vi "CAN Jaguar Config Limits.vi"(6 "Reverse Limit Position":dbl, 8 "error in (no error)":errorcluster, 9 "Forward Limit Position":dbl, 10 "Limit Mode":T1, 11 "CAN Jaguar Ref":T2={"Device Number"=0, "Control Mode"=enum."Percent VBus", "Inverted"=FALSE, "Semaphore"=refnum, "Max Vout"=12.0, "DevStatus"={"status"=FALSE, "code"=0, "source"=""}}) -> (0 "error out":errorcluster, 3 "CAN Jaguar Ref Out":T2={"Device Number"=0, "Control Mode"=enum."Percent VBus", "Inverted"=FALSE, "Semaphore"=refnum, "Max Vout"=12.0, "DevStatus"={"status"=FALSE, "code"=0, "source"=""}})   [LabVIEW 2009, in "CAN.lvlib"]
uses:
  CAN.lvlib
  SubVIs/CAN Motor Message IDs.ctl
  SubVIs/CAN Jaguar Control Mode.ctl
  SubVIs/CAN Jaguar Ref.ctl
  SubVIs/CAN Jaguar Limit Mode.ctl
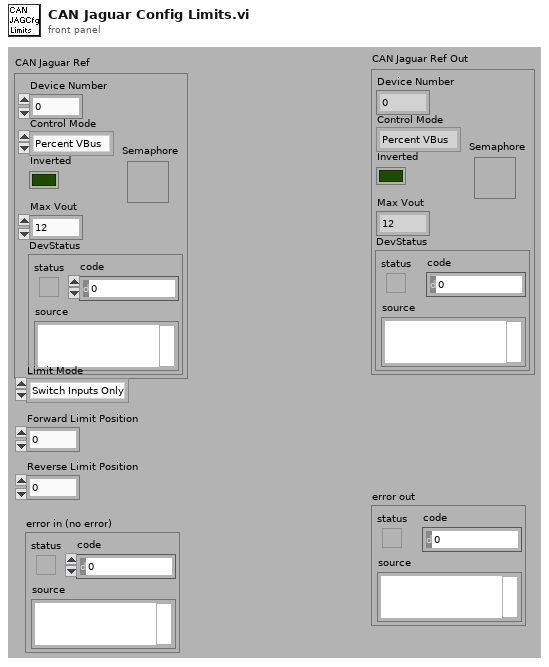
[diagram p1: front panel]
types:
  T1 = typedef "CAN.lvlib/CAN Jaguar Limit Mode.ctl" = enum16{"Switch Inputs Only", "Soft Position Limits"}
  T2 = typedef "CAN.lvlib/CAN Jaguar Ref.ctl" = cluster{"Device Number":u8, "Control Mode":T3, "Inverted":bool, "Semaphore":T4, "Max Vout":dbl, "DevStatus":errorcluster}
  T3 = typedef "CAN.lvlib/CAN Jaguar Control Mode.ctl" = enum16{"Percent VBus", "Speed", "Position", "Current"}
  T4 = typedef "Semaphore RefNum" = refnum<k1>
  T5 = enum16{"big-endian, network order", "native, host order", "little-endian"}
  T6 = typedef "CAN.lvlib/CAN Motor Message IDs.ctl" = u32
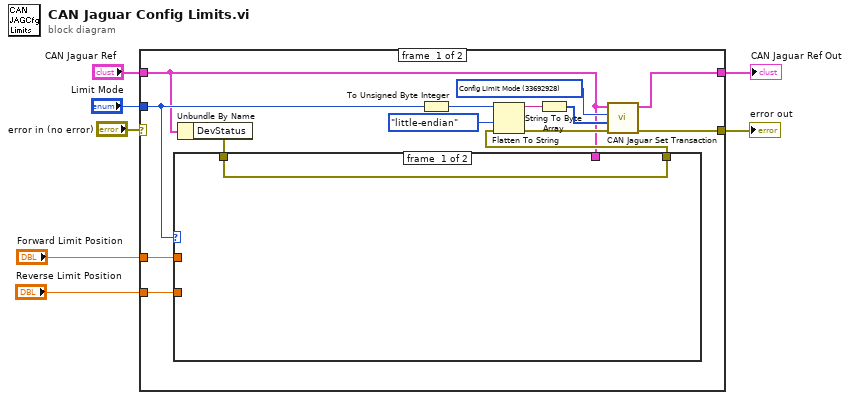
[diagram p0: block diagram]
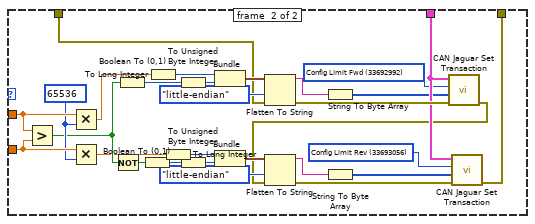
[diagram p2: hidden frame]
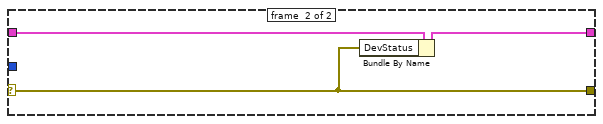
[diagram p3: hidden frame]
diagram:
  n1 = case shown="No Error" "error in (no error)" {
    selector: "error in (no error)" -> [_ w52]
    tunnel: [w11 w52] -> w7
    tunnel: [w12 w53] -> w5
    tunnel: "CAN Jaguar Ref" -> [w8 w54]
    tunnel: "Limit Mode" -> [w18 _]
    tunnel: "Forward Limit Position" -> [w17 _]
    tunnel: "Reverse Limit Position" -> [w16 _]
    frame #0 {
      w9 = T6 33692928 items=["Volt Enable"=33685504, "Volt Disable"=33685568, "Volt Set"=33685632, "Volt Set Ramp"=33685696, "Speed Enable"=33686528, "Speed Disable"=33686592, "Speed Set"=33686656, "Speed P"=33686720, "Speed I"=33686784, "Speed D"=33686848, "Speed Ref"=33686912, "Position Enable"=33688576, "Position Disable"=33688640, "Position Set"=33688704, "Position P"=33688768, "Position I"=33688832, "Position D"=33688896, "Position Ref"=33688960, "Current Enable"=33689600, "Current Disable"=33689664, "Current Set"=33689728, "Current P"=33689792, "Current I"=33689856, "Current D"=33689920, "Status VOut"=33690624, "Status VBus"=33690688, "Status Current"=33690752, "Status Temp"=33690816, "Status Position"=33690880, "Status Speed"=33690944, "Status Limit"=33691008, "Status Fault"=33691072, "Status Power"=33691136, "Config Num Brushes"=33692672, "Config Encoder Lines"=33692736, "Config Pot Turns"=33692800, "Config Brake Coast"=33692864, "Config Limit Mode"=33692928, "Config Limit Fwd"=33692992, "Config Limit Rev"=33693056, "Config Max VOut"=33693120, "Config Fault Time"=33693184, "Motor Ack"=33693696] ("CAN Motor Message IDs")
      n2 = Unbundle By Name(w8) -> ("DevStatus"=w14:errorcluster)
      n3 = case shown="\"Soft Position Limits\"" w18 {
        tunnel: w17 -> [_ w48]
        tunnel: w16 -> [_ w47]
        tunnel: w14 -> [w22 w40]
        tunnel: [w22 w27] -> w15
        tunnel: w8 -> [_ w30]
        frame #0 {
        }
        frame #1 {
          w23 = T6 33693056 items=["Volt Enable"=33685504, "Volt Disable"=33685568, "Volt Set"=33685632, "Volt Set Ramp"=33685696, "Speed Enable"=33686528, "Speed Disable"=33686592, "Speed Set"=33686656, "Speed P"=33686720, "Speed I"=33686784, "Speed D"=33686848, "Speed Ref"=33686912, "Position Enable"=33688576, "Position Disable"=33688640, "Position Set"=33688704, "Position P"=33688768, "Position I"=33688832, "Position D"=33688896, "Position Ref"=33688960, "Current Enable"=33689600, "Current Disable"=33689664, "Current Set"=33689728, "Current P"=33689792, "Current I"=33689856, "Current D"=33689920, "Status VOut"=33690624, "Status VBus"=33690688, "Status Current"=33690752, "Status Temp"=33690816, "Status Position"=33690880, "Status Speed"=33690944, "Status Limit"=33691008, "Status Fault"=33691072, "Status Power"=33691136, "Config Num Brushes"=33692672, "Config Encoder Lines"=33692736, "Config Pot Turns"=33692800, "Config Brake Coast"=33692864, "Config Limit Mode"=33692928, "Config Limit Fwd"=33692992, "Config Limit Rev"=33693056, "Config Max VOut"=33693120, "Config Fault Time"=33693184, "Motor Ack"=33693696] ("CAN Motor Message IDs")
          w46 = 65536
          w26 = T6 33692992 items=["Volt Enable"=33685504, "Volt Disable"=33685568, "Volt Set"=33685632, "Volt Set Ramp"=33685696, "Speed Enable"=33686528, "Speed Disable"=33686592, "Speed Set"=33686656, "Speed P"=33686720, "Speed I"=33686784, "Speed D"=33686848, "Speed Ref"=33686912, "Position Enable"=33688576, "Position Disable"=33688640, "Position Set"=33688704, "Position P"=33688768, "Position I"=33688832, "Position D"=33688896, "Position Ref"=33688960, "Current Enable"=33689600, "Current Disable"=33689664, "Current Set"=33689728, "Current P"=33689792, "Current I"=33689856, "Current D"=33689920, "Status VOut"=33690624, "Status VBus"=33690688, "Status Current"=33690752, "Status Temp"=33690816, "Status Position"=33690880, "Status Speed"=33690944, "Status Limit"=33691008, "Status Fault"=33691072, "Status Power"=33691136, "Config Num Brushes"=33692672, "Config Encoder Lines"=33692736, "Config Pot Turns"=33692800, "Config Brake Coast"=33692864, "Config Limit Mode"=33692928, "Config Limit Fwd"=33692992, "Config Limit Rev"=33693056, "Config Max VOut"=33693120, "Config Fault Time"=33693184, "Motor Ack"=33693696] ("CAN Motor Message IDs")
          n4 = Greater?(x=w48, y=w47) -> (0:w41:bool)
          n5 = Multiply(x=w48, y=w46) -> (x*y=w44:dbl)
          n6 = Multiply(x=w47, y=w46) -> (x*y=w33:dbl)
          n7 = Not(x=w41) -> (.not. x?=w32:bool)
          n8 = Boolean To (0,1)(Boolean=w41) -> (0, 1=w43:i16)
          n9 = Boolean To (0,1)(Boolean=w32) -> (0, 1=w38:i16)
          n10 = To Long Integer(number=w44) -> (32bit integer=w45:i32)
          n11 = To Long Integer(number=w33) -> (32bit integer=w37:i32)
          n12 = To Unsigned Byte Integer(number=w43) -> (unsigned 8bit integer=w42:u8)
          n13 = To Unsigned Byte Integer(number=w38) -> (unsigned 8bit integer=w39:u8)
          n14 = Bundle(w45, w42) -> (w49:cluster{i32, u8})  [unwired: 1 out]
          n15 = Bundle(w37, w39) -> (w36:cluster{i32, u8})  [unwired: 1 out]
          n16 = Flatten To String(anything=w49, byte order (0:big-endian, network order)=T5."little-endian", error in (no error)=w40) -> (data string=w51:string, error out=w31:errorcluster)  [unwired: 2 out]
          n17 = String To Byte Array(string=w51) -> (unsigned byte array=w25:u8[])
          n18 = call "CAN Jaguar Set Transaction.vi"("error in"=w31, "Data"=w25, "Message ID"=w26, "CAN Jaguar Ref"=w30) -> ("error out"=w29:errorcluster)  [unwired: 7 out]
          n19 = Flatten To String(anything=w36, byte order (0:big-endian, network order)=T5."little-endian", error in (no error)=w29) -> (data string=w34:string, error out=w28:errorcluster)  [unwired: 2 out]
          n20 = String To Byte Array(string=w34) -> (unsigned byte array=w24:u8[])
          n21 = call "CAN Jaguar Set Transaction.vi"("error in"=w28, "Data"=w24, "Message ID"=w23, "CAN Jaguar Ref"=w30) -> ("error out"=w27:errorcluster)  [unwired: 7 out]
        }
      }
      n22 = To Unsigned Byte Integer(number=w18) -> (unsigned 8bit integer=w19:u8)
      n23 = Flatten To String(anything=w19, byte order (0:big-endian, network order)=T5."little-endian", error in (no error)=w15) -> (data string=w20:string, error out=w13:errorcluster)  [unwired: 2 out]
      n24 = String To Byte Array(string=w20) -> (unsigned byte array=w10:u8[])
      n25 = call "CAN Jaguar Set Transaction.vi"("error in"=w13, "Data"=w10, "Message ID"=w9, "CAN Jaguar Ref"=w8) -> ("error out"=w11:errorcluster, "CAN Jaguar Ref Out"=w12:T2)  [unwired: 6 out]
    }
    frame #1 {
      n26 = Bundle By Name(cluster=w54, "DevStatus"=w52) -> (w53:T2)
    }
  }
  "CAN Jaguar Ref Out" <- w5
  "error out" <- w7
